vi "SetupImaqTrigger.vi"(0 "IMAQ Session In":refnum<k11>, 1 "error in (no error)":errorcluster) -> (2 "IMAQ Session Out":refnum<k11>, 3 "Trigger status":bool, 4 "error out":errorcluster)   [LabVIEW 2012]
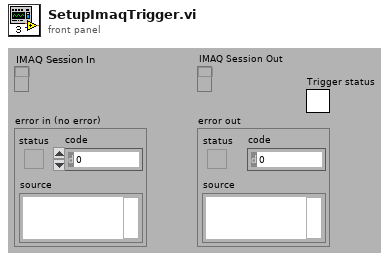
[diagram p1: front panel]
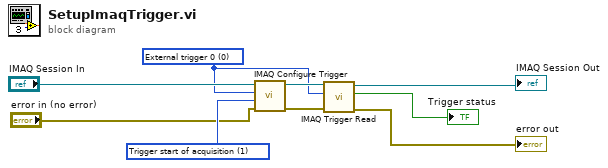
[diagram p0: block diagram]
diagram:
  w4 = u32 0 items=["External trigger 0", "External trigger 1", "External trigger 2", "External trigger 3", "RTSI line 0", "RTSI line 1", "RTSI line 2", "RTSI line 3", "RTSI line 4", "RTSI line 5", "RTSI line 6"] ("Trigger line")
  w9 = u32 1 items=["Disabled", "Trigger start of acquisition", "Trigger start of each buffer list", "Trigger each buffer", "Trigger each line (linescan)"] ("Trigger action")
  n1 = call <vilib>:"IMAQ Configure Trigger.vi"("error in (no error)"="error in (no error)", "Trigger action"=w9, "Trigger line"=w4, "IMAQ Session In"="IMAQ Session In") -> ("error out"=w5:errorcluster, "IMAQ Session Out"=w6:refnum<k11>)  [unwired: 6 in]
  n2 = call <vilib>:"IMAQ Trigger Read.vi"("error in (no error)"=w5, "Trigger line"=w4, "IMAQ Session In"=w6) -> ("error out"=→"error out":errorcluster, "Trigger status"=→"Trigger status":bool, "IMAQ Session Out"=→"IMAQ Session Out":refnum<k11>)  [unwired: 6 in]
